vi "Set Asymmetry Curve.vi"(7 "SigScale":dbl, 8 "error in (no error)":errorcluster caption="错误输入（无错误）", 9 "NumPoints":i32, 10 "AsymArray":dbl, 11 "asicHandle":i32) -> (0 "error out":errorcluster caption="错误输出", 2 "AsymArray out":dbl, 3 "function return":i32)   [LabVIEW 2018]
doc: "extern int __stdcall APSxSetAsymmetryCurve (int asicHandle, IN double * AsymArray, IN int NumPoints, IN double SigScale);"
uses:
  APSx.dll/APSx.dll
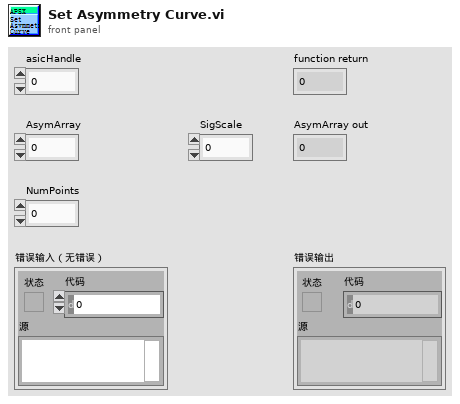
[diagram p1: front panel]
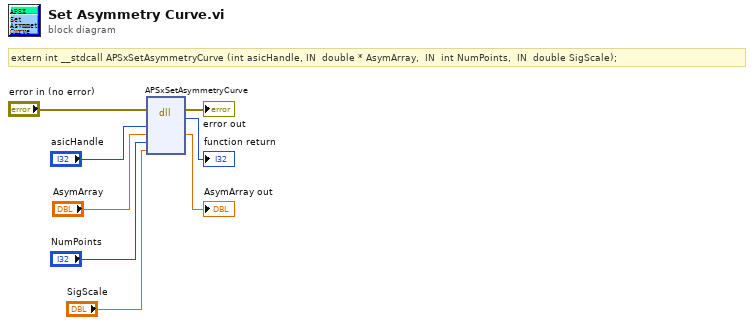
[diagram p0: block diagram]
diagram:
  # "extern int __stdcall APSxSetAsymmetryCurve (int asicHandle, IN  double * AsymArray,  IN  int NumPoints,  IN  double SigScale);"
  n1 = dll-call lib="PTH2[abs D项目Feng恒隆项目Labview传感器对中台SourcesAPSx.dllAPSx.*" fn="APSxSetAsymmetryCurve"(error in="error in (no error)", "asicHandle"="asicHandle", "AsymArray"="AsymArray", "NumPoints"="NumPoints", "SigScale"="SigScale") -> (error out=→"error out":errorcluster, →"function return":i32, "AsymArray"=→"AsymArray out":dbl)  [unwired: 5 in, 1 out]
